vi "Get New Level.vi"(8 "error in (no error)":errorcluster, 11 "Water Level in":refnum<class "Water Level.lvclass">) -> (0 "error out":errorcluster, 2 "Level":dbl, 3 "Water Level out":refnum<class "Water Level.lvclass">)   [LabVIEW 2018, in "Water Level.lvlib" / "Water Level.lvclass"]
doc: "Child classes should NOT override this VI. Any functionality a child class would add should instead be added by overriding Get Water Level.vi."
uses:
  Water Level.lvclass
  C:/Program Files (x86)/National Instruments/LabVIEW 2018/vi.lib/ActorFramework/Actor/Actor.lvclass
  <vilib>/ActorFramework/Actor/Actor.lvclass/Actor.ctl
  Water Level.lvclass/Water Level.ctl
  Update Water Level Msg/Update Water Level Msg.lvclass
  <vilib>/ActorFramework/Actor/Actor.lvclass
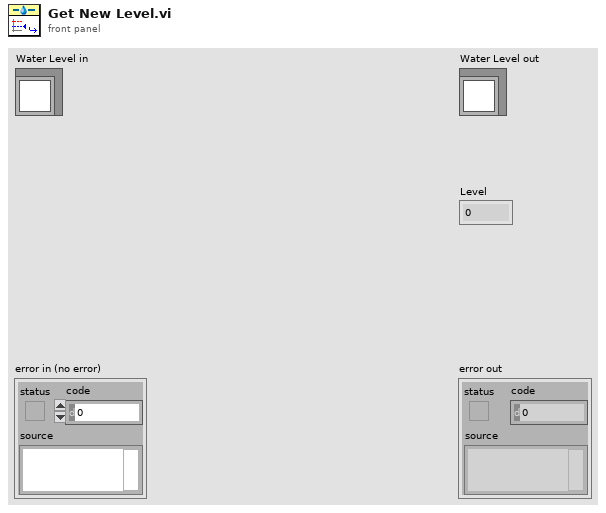
[diagram p1: front panel]
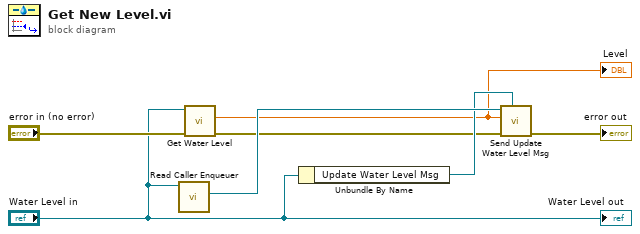
[diagram p0: block diagram]
diagram:
  n1 = call <vilib>:"Read Caller Enqueuer.vi"("Actor"="Water Level in") -> ("Caller Enqueuer"=w6:refnum<class "Message Enqueuer.lvclass">)  [unwired: 10 in]
  n2 = call-dynamic "Get Water Level.vi"("error in (no error)"="error in (no error)", "Water Level in"="Water Level in") -> ("error out"=w4:errorcluster, "Water Level"=w1:dbl)  [unwired: 8 in]
  "Level" <- w1
  n3 = Unbundle By Name("Water Level in") -> ("Update Water Level Msg"=w5:refnum<class "Update Water Level Msg.lvclass">)
  n4 = call "Send Update Water Level Msg.vi"("Update Water Level Msg"=w5, "error in (no error)"=w4, "Water Level"=w1, "Message Enqueuer"=w6) -> ("error out"=→"error out":errorcluster)  [unwired: 7 in]
  "Water Level out" <- "Water Level in"
